vi "Serrure numérique.vi"() -> ()   [LabVIEW 2018]
panel:
  out "Boolean":bool
  in  "Bouton3":i8(knob) scale=0.0..9.0
  in  "Bouton1":i8(knob) min=0 max=9 scale=0.0..9.0
  in  "Bouton2":i8(knob) scale=0.0..9.0
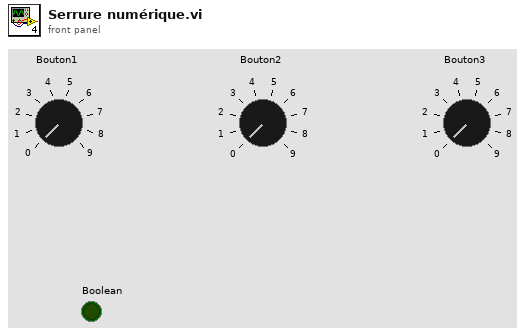
[diagram p1: front panel]
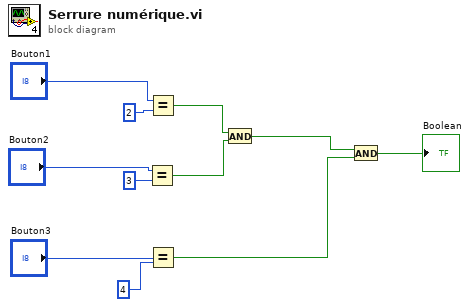
[diagram p0: block diagram]
diagram:
  n1 = Equal?(x="Bouton2", y=i8 3) -> (x = y?=w4:bool)
  n2 = Equal?(x="Bouton1", y=i8 2) -> (x = y?=w5:bool)
  n3 = Equal?(x="Bouton3", y=i8 4) -> (x = y?=w3:bool)
  n4 = And(x=w5, y=w4) -> (x .and. y?=w2:bool)
  n5 = And(x=w2, y=w3) -> (x .and. y?=→"Boolean":bool)
